vi "Two Button Dialog with Timeout.vi"(0 "message":string, 1 "T Timeout(-1 s)":i32=-1, 2 "T button name (\"OK\")":string="OK", 3 "F button name (\"Cancel\")":string="Cancel", 4 "F Timeout(-1 s)":i32=-1) -> (5 "T button?":bool)   [LabVIEW 2017]
uses:
  a539abf7-d72e-4e1a-867b-c48a8ed28406.vi
  a000c3c0-17f0-4be0-b5ae-7b04c78b6241.vi
  7f025491-3c73-41eb-90d8-dc68797bdda8.vi
panel:
  out "font":T1
  in  "Cancel":bool
  in  "OK":bool
  out "String":string
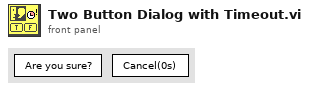
[diagram p1: front panel]
types:
  T1 = cluster{"Font Name:":string, "Size":i16, "Strikeout?":bool, "Italic?":bool, "Underline?":bool, "Outline?":bool, "Shadow?":bool, "Bold?":bool}
  T2 = typedef "LVFontTypeDef.ctl" = cluster{"Font Name":string, "Size":u16, "Bold":bool, "Italic":bool, "Underline":bool, "Strikeout":bool, "Color":u32}
  T3 = cluster{"left":i16, "top":i16, "right":i16, "bottom":i16}
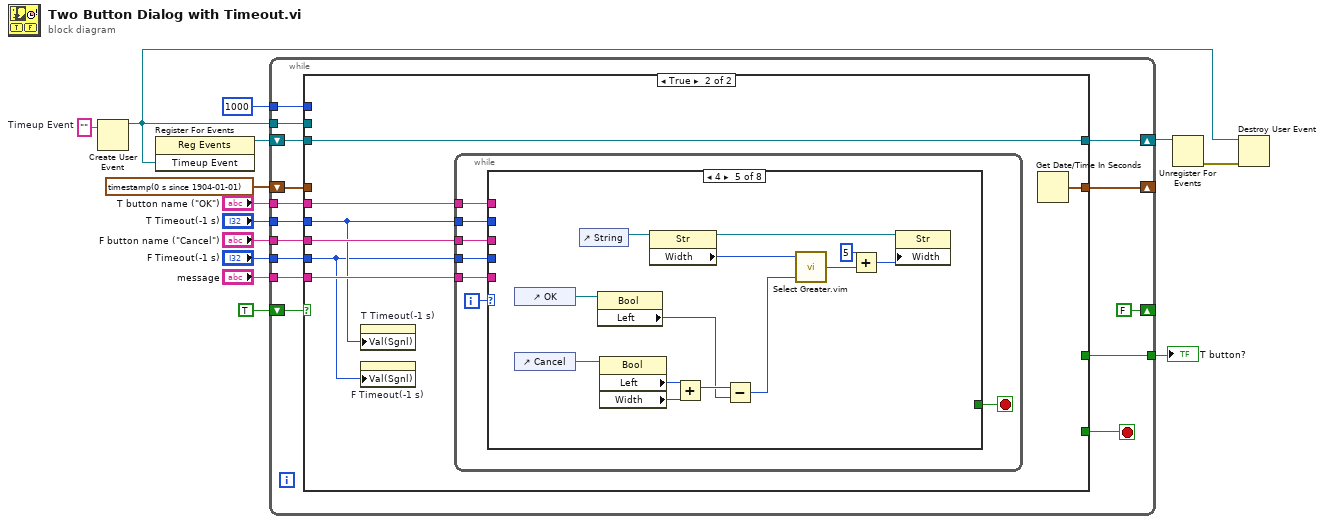
[diagram p0: block diagram]
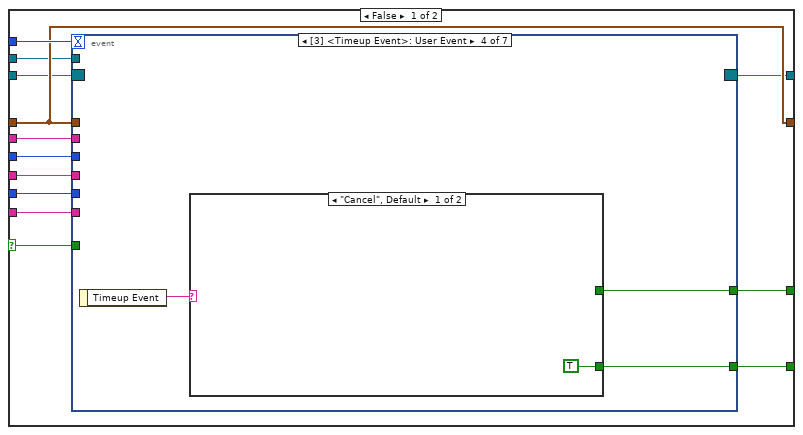
[diagram p2: hidden frame]
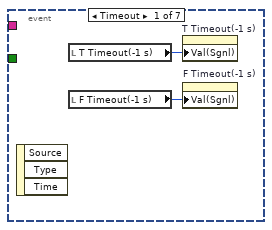
[diagram p3: hidden frame]
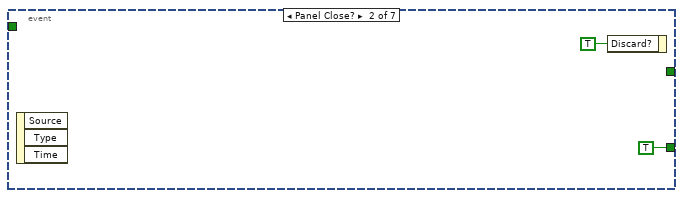
[diagram p4: hidden frame]
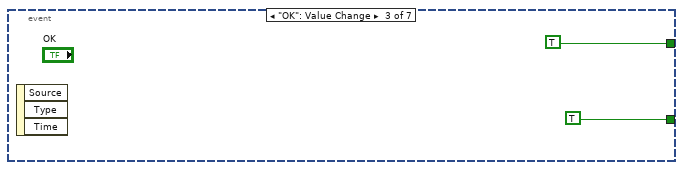
[diagram p5: hidden frame]
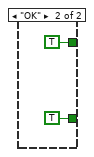
[diagram p6: hidden frame]
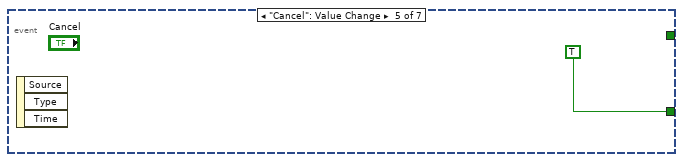
[diagram p7: hidden frame]
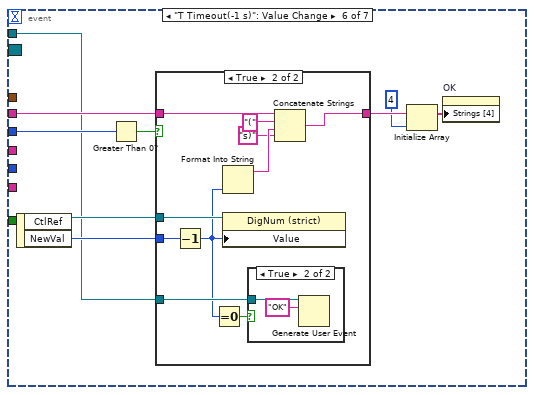
[diagram p8: hidden frame]
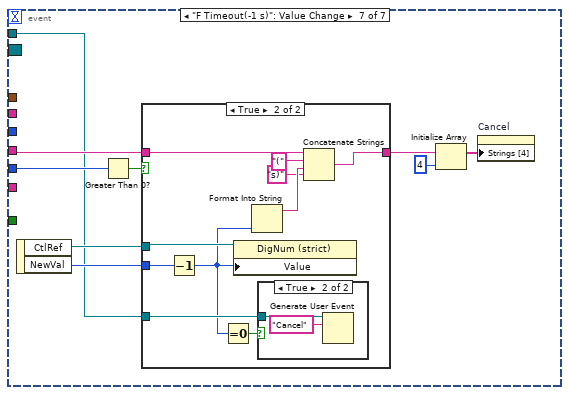
[diagram p11: hidden frame]
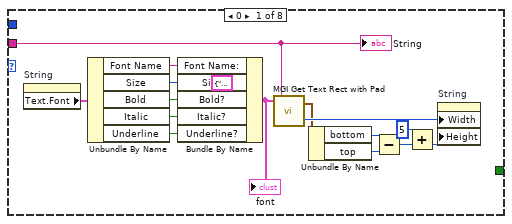
[diagram p14: hidden frame]
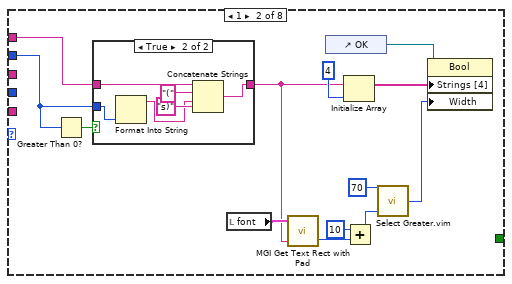
[diagram p15: hidden frame]
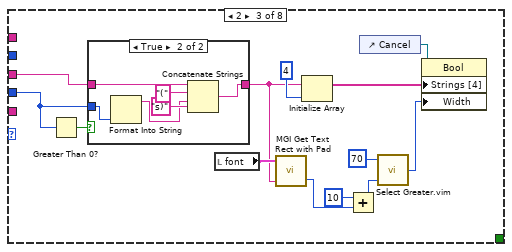
[diagram p17: hidden frame]
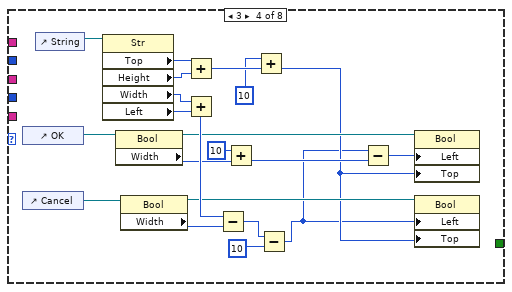
[diagram p19: hidden frame]
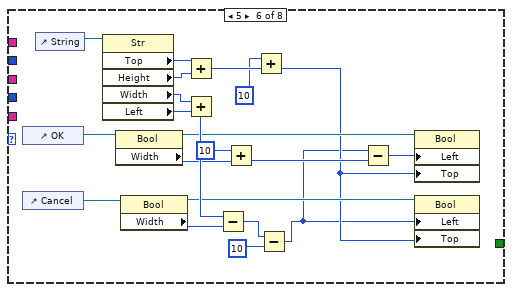
[diagram p20: hidden frame]
diagram:
  w5 = ""  # Timeup Event
  n1 = Create User Event(user event datatype=w5) -> (user event=w1:refnum<user-event>)  [unwired: 1 in, 1 out]
  n2 = register-events(w1) -> (reference out=w4:refnum<event-registration>)  [unwired: 2 in, 1 out]
  n3 = while {
    tunnel: [w28] -> w14
    tunnel: "T button name (\"OK\")" -> [w24]
    tunnel: "F button name (\"Cancel\")" -> [w22]
    tunnel: "message" -> [w25]
    shift-right: [FALSE] -> _
    shift-left: TRUE -> [w27]
    tunnel: "F Timeout(-1 s)" -> [w21]
    tunnel: "T Timeout(-1 s)" -> [w23]
    shift-right: [w20] -> _
    shift-left: timestamp(0 s since 1904-01-01) ("seconds since 1Jan1904") -> [w19]
    tunnel: 1000 -> [w18]
    shift-right: [w16] -> w3
    shift-left: w4 -> [w17]
    tunnel: w1 -> [w15]
    stop <- w29 stop-if-true
    n4 = case shown="True" w27 {
      selector: w27 -> [w39 _]
      tunnel: [w42 _] -> w29
      tunnel: [w41 _] -> w28
      tunnel: w18 -> [w40 _]
      tunnel: w25 -> [w34 w104]
      tunnel: w24 -> [w38 w102]
      tunnel: w23 -> [w37 w101]
      tunnel: w22 -> [w36 w103]
      tunnel: w21 -> [w35 w100]
      tunnel: [w33 w106] -> w20
      tunnel: w19 -> [w33 _]
      tunnel: w17 -> [w32 w105]
      tunnel: [w31 w105] -> w16
      tunnel: w15 -> [w30 _]
      frame False {
        n5 = event shown="[3] <Timeup Event>: User Event" {
          selector: w32 -> [_ _ _ _ _ _ _]
          dyn-events: [_ _ _ _ _ _ _] -> w31
          timeout: w40 -> [_ _ _ _ _ _ _]
          tunnel: [_ TRUE ("Discard?") TRUE ("Discard?") w50 TRUE ("Discard?") _ _] -> w42
          tunnel: [_ _ TRUE w49 _ _ _] -> w41
          tunnel: w39 -> [_ _ _ _ _ _ _]
          tunnel: w38 -> [_ _ _ _ _ w64 _]
          tunnel: w37 -> [_ _ _ _ _ w62 _]
          tunnel: w36 -> [_ _ _ _ _ _ w82]
          tunnel: w35 -> [_ _ _ _ _ _ w81]
          tunnel: w34 -> [_ _ _ _ _ _ _]
          tunnel: w33 -> [_ _ _ _ _ _ _]
          tunnel: w30 -> [_ _ _ _ _ w56 w78]
          event Timeout {
            n6 = event-data() -> ()  [unwired: 1 in, 3 out]
            n7 = local read "T Timeout(-1 s)"() -> (w43:i32)
            n8 = local read "F Timeout(-1 s)"() -> (w44:i32)
            n9 = property on="T Timeout(-1 s)" class="DigNum (strict)"("Val(Sgnl)"=w43) -> ()  [unwired: 2 in, 2 out]
            n10 = property on="F Timeout(-1 s)" class="DigNum (strict)"("Val(Sgnl)"=w44) -> ()  [unwired: 2 in, 2 out]
          }
          event Panel Close? {
            n11 = event-data() -> ()  [unwired: 1 in, 3 out]
            n12 = event-data("Discard?"=TRUE) -> ()  [unwired: 1 in, 1 out]
          }
          event "OK": Value Change {
            n13 = event-data() -> ()  [unwired: 1 in, 3 out]
          }
          event User Event {
            n14 = event-data() -> ("Timeup Event"=w51:string)  [unwired: 1 in]
            n15 = case shown="\"Cancel\", Default" w51 {
              tunnel: [TRUE ("Discard?") TRUE ("Discard?")] -> w50
              tunnel: [_ TRUE ("Discard?")] -> w49
              frame "Cancel", Default {
              }
              frame "OK" {
              }
            }
          }
          event "Cancel": Value Change {
            n16 = event-data() -> ()  [unwired: 1 in, 3 out]
          }
          event "T Timeout(-1 s)": Value Change {
            n17 = event-data() -> ("CtlRef"=w58:refnum<vi>, "NewVal"=w57:i32)  [unwired: 1 in]
            n18 = Greater Than 0?(x=w62) -> (x > 0?=w63:bool)
            n19 = case shown="True" w63 {
              tunnel: w64 -> [w65 w75]
              tunnel: [w65 w71] -> w61
              tunnel: w57 -> [_ w70]
              tunnel: w58 -> [_ w69]
              tunnel: w56 -> [_ w67]
              frame False {
              }
              frame True {
                n20 = Decrement(x=w70) -> (x-1=w66:i32)
                n21 = Equal To 0?(x=w66) -> (x = 0?=w68:bool)
                n22 = Format Into String(w66) -> (resulting string=w74:string)  [unwired: 3 in, 1 out]
                n23 = property class="DigNum (strict)"(reference=w69, "Value"=w66) -> ()  [unwired: 1 in, 2 out]
                n24 = case shown="True" w68 {
                  tunnel: w67 -> [_ w77]
                  frame False {
                  }
                  frame True {
                    n25 = Generate User Event(user event=w77, event data cluster="OK" ("event data")) -> ()  [unwired: 2 in, 2 out]
                  }
                }
                n26 = Concatenate Strings(w75, "(" ("string"), w74, "s)" ("string")) -> (w71:string)
              }
            }
            n27 = Initialize Array(w61, 4 ("dimension size")) -> (w60:string[])
            n28 = property on="OK" class="Bool"("Strings [4]"=w60) -> ()  [unwired: 2 in, 2 out]
          }
          event "F Timeout(-1 s)": Value Change {
            n29 = event-data() -> ("CtlRef"=w80:refnum<vi>, "NewVal"=w79:i32)  [unwired: 1 in]
            n30 = Greater Than 0?(x=w81) -> (x > 0?=w86:bool)
            n31 = case shown="True" w86 {
              tunnel: w82 -> [w87 w97]
              tunnel: [w87 w93] -> w85
              tunnel: w79 -> [_ w92]
              tunnel: w80 -> [_ w91]
              tunnel: w78 -> [_ w89]
              frame False {
              }
              frame True {
                n32 = Decrement(x=w92) -> (x-1=w88:i32)
                n33 = Equal To 0?(x=w88) -> (x = 0?=w90:bool)
                n34 = property class="DigNum (strict)"(reference=w91, "Value"=w88) -> ()  [unwired: 1 in, 2 out]
                n35 = Format Into String(w88) -> (resulting string=w96:string)  [unwired: 3 in, 1 out]
                n36 = case shown="True" w90 {
                  tunnel: w89 -> [_ w99]
                  frame False {
                  }
                  frame True {
                    n37 = Generate User Event(user event=w99, event data cluster="Cancel" ("event data")) -> ()  [unwired: 2 in, 2 out]
                  }
                }
                n38 = Concatenate Strings(w97, "(" ("string"), w96, "s)" ("string")) -> (w93:string)
              }
            }
            n39 = Initialize Array(w85, 4 ("dimension size")) -> (w84:string[])
            n40 = property on="Cancel" class="Bool"("Strings [4]"=w84) -> ()  [unwired: 2 in, 2 out]
          }
        }
      }
      frame True {
        n41 = property on="T Timeout(-1 s)" class="DigNum (strict)"("Val(Sgnl)"=w101) -> ()  [unwired: 2 in, 2 out]
        n42 = property on="F Timeout(-1 s)" class="DigNum (strict)"("Val(Sgnl)"=w100) -> ()  [unwired: 2 in, 2 out]
        n43 = while {
          tunnel: w104 -> [w113]
          tunnel: w103 -> [w110]
          tunnel: w102 -> [w109]
          tunnel: w101 -> [w108]
          tunnel: w100 -> [w107]
          i -> [w112]
          stop <- w111 stop-if-true
          n44 = case shown="4" w112 {
            tunnel: w113 -> [w128 _ _ _ _ _ _ _]
            tunnel: [_ _ _ _ _ _ _ TRUE] -> w111
            tunnel: w110 -> [_ _ w158 _ _ _ _ _]
            tunnel: w109 -> [_ w139 _ _ _ _ _ _]
            tunnel: w108 -> [_ w138 _ _ _ _ _ _]
            tunnel: w107 -> [_ _ w157 _ _ _ _ _]
            frame 0 {
              n45 = property on="String" class="Str"() -> ("Text.Font"=w129:T2)  [unwired: 2 in, 2 out]
              n46 = Unbundle By Name(w129) -> ("Font Name"=w125:string, "Size"=w124:u16, "Bold"=w123:bool, "Italic"=w121:bool, "Underline"=w122:bool)
              n47 = Bundle By Name(cluster=T1 {"Font Name:"="", "Size"=0, "Strikeout?"=FALSE, "Italic?"=FALSE, "Underline?"=FALSE, "Outline?"=FALSE, "Shadow?"=FALSE, "Bold?"=FALSE} ("Font"), "Font Name:"=w125, "Size"=w124, "Bold?"=w123, "Italic?"=w121, "Underline?"=w122) -> (w126:T1)
              "font" <- w126
              n48 = call <userlib>:"MGI Get Text Rect with Pad.vi"("Text"=w128, "Font"=w126) -> ("Width"=w120:i16, "Rect"=w119:T3)  [unwired: 1 in]
              n49 = Unbundle By Name(w119) -> ("bottom"=w116:i16, "top"=w118:i16)
              n50 = Subtract(x=w116, y=w118) -> (x-y=w117:i16)
              n51 = Add(x=i16 5, y=w117) -> (x+y=w115:i16)
              n52 = property on="String" class="Str"("Width"=w120, "Height"=w115) -> ()  [unwired: 2 in, 2 out]
              "String" <- w128
            }
            frame 1 {
              n53 = Greater Than 0?(x=w138) -> (x > 0?=w142:bool)
              n54 = case shown="True" w142 {
                tunnel: w139 -> [w143 w149]
                tunnel: [w143 w146] -> w135
                tunnel: w138 -> [_ w144]
                frame False {
                }
                frame True {
                  n55 = Format Into String(w144) -> (resulting string=w145:string)  [unwired: 3 in, 1 out]
                  n56 = Concatenate Strings(w149, "(" ("string"), w145, "s)" ("string")) -> (w146:string)
                }
              }
              n57 = local read "font"() -> (w136:T1)
              n58 = call <userlib>:"MGI Get Text Rect with Pad.vi"("Text"=w135, "Font"=w136) -> ("Width"=w134:i16)  [unwired: 1 in, 1 out]
              n59 = control-ref of="OK"() -> (w137:refnum<vi>)
              n60 = Initialize Array(w135, 4 ("dimension size")) -> (w141:string[])
              n61 = Add(x=i16 10, y=w134) -> (x+y=w131:i16)
              n62 = call "Select Greater.vim"("A"=70, "B"=w131) -> ("lesser"=w130:i32)  [unwired: 3 in]
              n63 = property on="Property Node" class="Bool"(reference=w137, "Strings [4]"=w141, "Width"=w130) -> ()  [unwired: 1 in, 2 out]
            }
            frame 2 {
              n64 = Greater Than 0?(x=w157) -> (x > 0?=w162:bool)
              n65 = case shown="True" w162 {
                tunnel: w158 -> [w163 w169]
                tunnel: [w163 w166] -> w155
                tunnel: w157 -> [_ w164]
                frame False {
                }
                frame True {
                  n66 = Format Into String(w164) -> (resulting string=w165:string)  [unwired: 3 in, 1 out]
                  n67 = Concatenate Strings(w169, "(" ("string"), w165, "s)" ("string")) -> (w166:string)
                }
              }
              n68 = local read "font"() -> (w156:T1)
              n69 = call <userlib>:"MGI Get Text Rect with Pad.vi"("Text"=w155, "Font"=w156) -> ("Width"=w153:i16)  [unwired: 1 in, 1 out]
              n70 = Initialize Array(w155, 4 ("dimension size")) -> (w161:string[])
              n71 = Add(x=i16 10, y=w153) -> (x+y=w151:i16)
              n72 = control-ref of="Cancel"() -> (w159:refnum<vi>)
              n73 = call "Select Greater.vim"("A"=70, "B"=w151) -> ("lesser"=w150:i32)  [unwired: 3 in]
              n74 = property on="Property Node" class="Bool"(reference=w159, "Strings [4]"=w161, "Width"=w150) -> ()  [unwired: 1 in, 2 out]
            }
            frame 3 {
              n75 = control-ref of="OK"() -> (w181:refnum<vi>)
              n76 = control-ref of="Cancel"() -> (w183:refnum<vi>)
              n77 = control-ref of="String"() -> (w190:refnum<vi>)
              n78 = property class="Str"(reference=w190) -> ("Top"=w189:i32, "Height"=w188:u32, "Width"=w186:u32, "Left"=w185:i32)  [unwired: 1 in, 2 out]
              n79 = property class="Bool"(reference=w181) -> (reference out=w176:refnum<vi>, "Width"=w180:u32)  [unwired: 1 in, 1 out]
              n80 = property class="Bool"(reference=w183) -> (reference out=w175:refnum<vi>, "Width"=w182:u32)  [unwired: 1 in, 1 out]
              n81 = Add(x=w189, y=w188) -> (x+y=w187:u32)
              n82 = Add(x=w186, y=w185) -> (x+y=w184:u32)
              n83 = Subtract(x=w184, y=w182) -> (x-y=w171:u32)
              n84 = Add(x=u32 10, y=w180) -> (x+y=w179:u32)
              n85 = Add(x=u32 10, y=w187) -> (x+y=w174:u32)
              n86 = Subtract(x=w171, y=u32 10 ("x")) -> (x-y=w170:u32)
              n87 = Subtract(x=w170, y=w179) -> (x-y=w177:u32)
              n88 = property class="Bool"(reference=w176, "Left"=w177, "Top"=w174) -> ()  [unwired: 1 in, 2 out]
              n89 = property class="Bool"(reference=w175, "Left"=w170, "Top"=w174) -> ()  [unwired: 1 in, 2 out]
            }
            frame 4 {
              n90 = control-ref of="OK"() -> (w201:refnum<vi>)
              n91 = control-ref of="Cancel"() -> (w202:refnum<vi>)
              n92 = control-ref of="String"() -> (w203:refnum<vi>)
              n93 = property class="Bool"(reference=w201) -> ("Left"=w196:i32)  [unwired: 1 in, 2 out]
              n94 = property class="Bool"(reference=w202) -> ("Left"=w198:i32, "Width"=w199:u32)  [unwired: 1 in, 2 out]
              n95 = property class="Str"(reference=w203) -> (reference out=w200:refnum<vi>, "Width"=w193:u32)  [unwired: 1 in, 1 out]
              n96 = Add(x=w198, y=w199) -> (x+y=w197:u32)
              n97 = Subtract(x=w197, y=w196) -> (x-y=w192:u32)
              n98 = call "Select Greater.vim"("A"=w193, "B"=w192) -> ("lesser"=w191:u32)  [unwired: 3 in]
              n99 = Add(x=i16 5, y=w191) -> (x+y=w194:u32)
              n100 = property class="Str"(reference=w200, "Width"=w194) -> ()  [unwired: 1 in, 2 out]
            }
            frame 5 {
              n101 = control-ref of="OK"() -> (w215:refnum<vi>)
              n102 = control-ref of="Cancel"() -> (w217:refnum<vi>)
              n103 = control-ref of="String"() -> (w224:refnum<vi>)
              n104 = property class="Str"(reference=w224) -> ("Top"=w223:i32, "Height"=w222:u32, "Width"=w220:u32, "Left"=w219:i32)  [unwired: 1 in, 2 out]
              n105 = property class="Bool"(reference=w215) -> (reference out=w210:refnum<vi>, "Width"=w214:u32)  [unwired: 1 in, 1 out]
              n106 = property class="Bool"(reference=w217) -> (reference out=w209:refnum<vi>, "Width"=w216:u32)  [unwired: 1 in, 1 out]
              n107 = Add(x=w223, y=w222) -> (x+y=w221:u32)
              n108 = Add(x=w220, y=w219) -> (x+y=w218:u32)
              n109 = Subtract(x=w218, y=w216) -> (x-y=w205:u32)
              n110 = Add(x=u32 10, y=w214) -> (x+y=w213:u32)
              n111 = Add(x=u32 10, y=w221) -> (x+y=w208:u32)
              n112 = Subtract(x=w205, y=u32 10 ("x")) -> (x-y=w204:u32)
              n113 = Subtract(x=w204, y=w213) -> (x-y=w211:u32)
              n114 = property class="Bool"(reference=w210, "Left"=w211, "Top"=w208) -> ()  [unwired: 1 in, 2 out]
              n115 = property class="Bool"(reference=w209, "Left"=w204, "Top"=w208) -> ()  [unwired: 1 in, 2 out]
            }
            frame 6 {
              n116 = call "Fit VI window to Visible Content.vi"("border spacing (2 px)"=10) -> ("error out"=w227:errorcluster)  [unwired: 5 in, 1 out]
              n117 = call <userlib>:"MGI Center Callee in Caller.vi"("Error In"=w227) -> ("Error Out"=w226:errorcluster)  [unwired: 10 in]
              n118 = call <vilib>:"Clear Errors.vi"("error in (no error)"=w226) -> ()  [unwired: 5 in, 2 out]
            }
            frame Default {
            }
          }
        }
        n119 = Get Date/Time In Seconds() -> (seconds since 1Jan1904=w106:timestamp)
      }
    }
  }
  "T button?" <- w14
  n120 = Unregister For Events(event registration refnum=w3) -> (error out=w2:errorcluster)  [unwired: 1 in]
  n121 = Destroy User Event(user event=w1, error in=w2) -> ()  [unwired: 1 out]
